vi "Main Page.vi"(8 "error in (no error)":errorcluster, 11 "Node Ptr":T1 format="%.0x") -> (0 "error out":errorcluster)   [LabVIEW 2020, in "G5 Regatron Custom Device System Explorer.lvlib"]
uses:
  G5 Regatron Custom Device System Explorer.lvlib
  <vilib>/NI VeriStand/Custom Device API/Custom Device Item Ref.ctl
  Shared/Constants.vi
  <vilib>/NI VeriStand/Custom Device API/Set Item Property (String).vi
  <vilib>/NI VeriStand/Custom Device API/Get Item Property (String).vi
  <vilib>/NI VeriStand/Custom Device API/Custom Device API.lvlib
  Shared/G5 Regatron Custom Device Shared.lvlib
panel:
  in  "Regatron IP Address":string="000.000.000.000"
  out "Version":string
  in  "SHDocVw.IWebBrowser":refnum<k7>(container)
  in  "Specific Header":cluster{"Section Name":string}={"Section Name"="Custom Device Item Settings"}
  in  "General Header":cluster{"Section Name":string}={"Section Name"="General Custom Device Settings"}
  in  "Description":string
  in  "Name":string
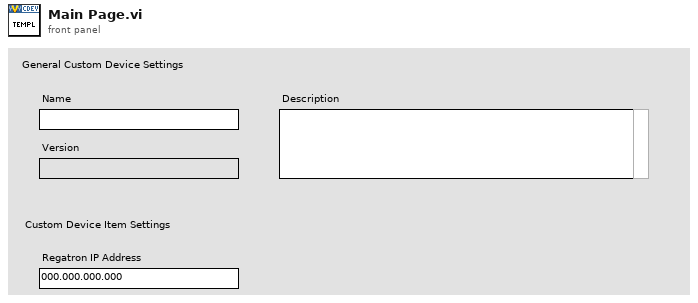
[diagram p1: front panel]
types:
  T1 = typedef "Custom Device API.lvlib/Custom Device Item Ref.ctl" = u64
  T2 = typedef "Custom Device API.lvlib/Custom Device Item Info.ctl" = cluster{"Name":string, "Is Channel":bool, "GUID":string, "Is Waveform":bool}
  T3 = typedef "Custom Device API.lvlib/Custom Device Commands.ctl" = enum16{"Default", "Item renamed", "Shutdown", "Dynamic button pressed"}
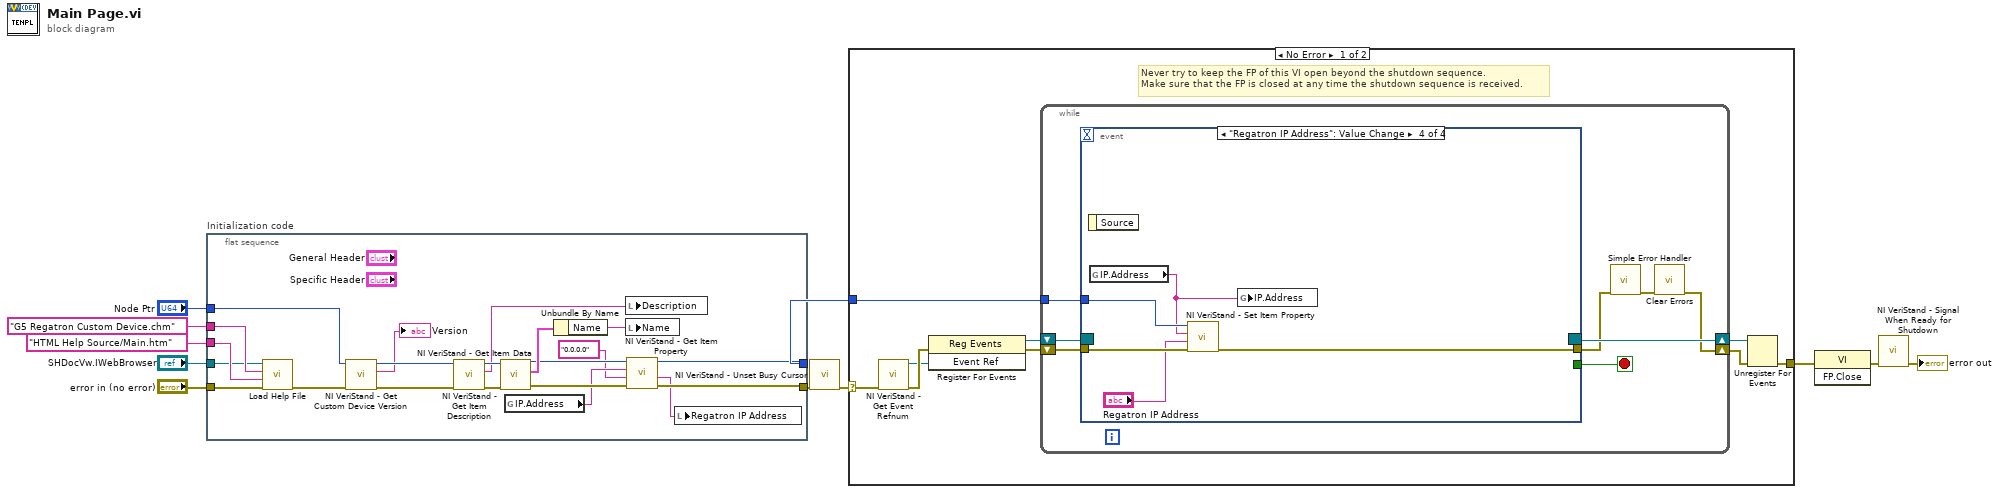
[diagram p0: block diagram]
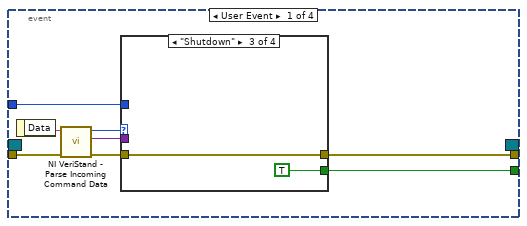
[diagram p2: hidden frame]
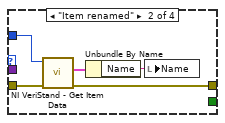
[diagram p4: hidden frame]
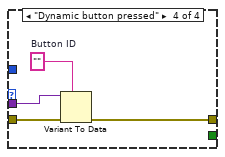
[diagram p5: hidden frame]
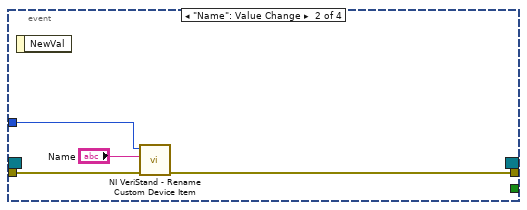
[diagram p6: hidden frame]
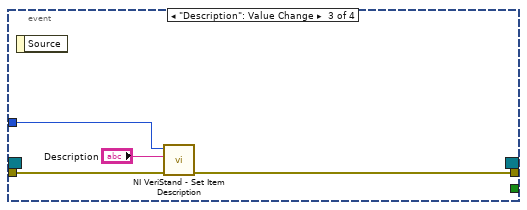
[diagram p7: hidden frame]
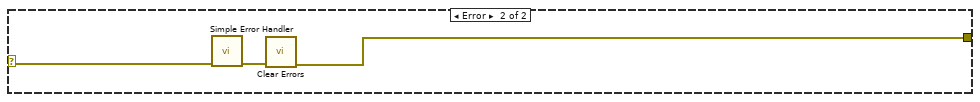
[diagram p8: hidden frame]
diagram:
  n1 = flat-sequence "Initialization code" {
    tunnel: "error in (no error)" -> [w23]
    tunnel: "Node Ptr" -> [w29]
    tunnel: [w16] -> w7
    tunnel: [w17] -> w4
    tunnel: "SHDocVw.IWebBrowser" -> [w19]
    tunnel: "HTML Help Source/Main.htm" ("HTML File") -> [w20]
    tunnel: "G5 Regatron Custom Device.chm" ("CD_CHM_FileName") -> [w21]
    frame #0 {
      n2 = call "Load Help File.vi"("error in (no error)"=w23, "HTML File to Load"=w20, "Main CHM File"=w21, "Browser"=w19) -> ("error out"=w22:errorcluster)  [unwired: 7 in]
      n3 = call <vilib>:"NI VeriStand - Get Custom Device Version.vi"("error in (no error)"=w22, "Device Ref in"=w29) -> ("error out"=w28:errorcluster, "Value"=→"Version":string, "Device Ref out"=w27:T1)  [unwired: 7 in]
      n4 = call <vilib>:"NI VeriStand - Get Item Description.vi"("error in (no error)"=w28, "Item Ref in"=w27) -> ("error out"=w31:errorcluster, "Description"=w24:string, "Item Ref out"=w32:T1)  [unwired: 7 out]
      n5 = call <vilib>:"NI VeriStand - Get Item Data.vi"("error in (no error)"=w31, "Item Ref in"=w32) -> ("error out"=w15:errorcluster, "Item Info"=w30:T2, "Item Ref out"=w18:T1)  [unwired: 7 out]
      n6 = global read "Constants.vi" "IP.Address"() -> (w14:string)
      n7 = Unbundle By Name(w30) -> ("Name"=w25:string)
      n8 = local write "Description"(w24) -> ()
      n9 = local write "Name"(w25) -> ()
      n10 = call-poly <vilib>:"NI VeriStand - Get Item Property.vi"("error in (no error)"=w15, "Default Value"="0.0.0.0", "Property Name"=w14, "Item Ref in"=w18) -> ("error out"=w16:errorcluster, "Value"=w12:string, "Item Ref out"=w17:T1)  [unwired: 4 in, 1 out]
      n11 = local write "Regatron IP Address"(w12) -> ()
    }
  }
  n12 = call <vilib>:"NI VeriStand - Unset Busy Cursor.vi"("error in (no error)"=w7) -> ("error out"=w6:errorcluster)  [unwired: 10 out]
  n13 = case shown="No Error" w6 {
    selector: w6 -> [w33 w85]
    tunnel: [w38 w83] -> w11
    tunnel: w4 -> [w34 _]
    frame No Error {
      # "Never try to keep the FP of this VI open beyond the shutdown sequence.\nMake sure that the FP is closed at any time the shutdown sequence is received."
      n14 = call <vilib>:"NI VeriStand - Get Event Refnum.vi"("error in (no error)"=w33) -> ("error out"=w41:errorcluster, "Event Ref"=w37:refnum<user-event>)  [unwired: 9 out]
      n15 = register-events(error in=w41, w37) -> (reference out=w35:refnum<event-registration>, error out=w36:errorcluster)  [unwired: 1 in]
      n16 = while {
        tunnel: w34 -> [w45]
        shift-right: [w42] -> w39
        shift-left: w36 -> [w48]
        shift-right: [w49] -> w40
        shift-left: w35 -> [w47]
        stop <- w46 stop-if-true
        n17 = event shown="[3] \"Regatron IP Address\": Value Change" {
          selector: w47 -> [_ _ _ _]
          dyn-events: [_ _ _ _] -> w49
          timeout: _ -> [_ _ _ _]
          tunnel: w48 -> [w57 w73 w76 w81]
          tunnel: [w53 _ _ _] -> w46
          tunnel: [w52 w72 w75 w79] -> w44
          tunnel: w45 -> [w51 w71 w77 w82]
          event User Event {
            n18 = event-data() -> ("Data"=w56:string)  [unwired: 1 out]
            n19 = call <vilib>:"NI VeriStand - Parse Incoming Command Data.vi"("error in (no error)"=w57, "Incoming data"=w56) -> ("error out"=w55:errorcluster, "Outgoing data"=w50:variant, "Action"=w54:T3)  [unwired: 7 out]
            n20 = case shown="\"Shutdown\"" w54 {
              tunnel: w55 -> [w58 w63 w64 w69]
              tunnel: [_ _ TRUE _] -> w53
              tunnel: [w58 w60 w64 w66] -> w52
              tunnel: w51 -> [_ w62 _ _]
              tunnel: w50 -> [_ _ _ w68]
              frame "Default", Default {
              }
              frame "Item renamed" {
                n21 = call <vilib>:"NI VeriStand - Get Item Data.vi"("error in (no error)"=w63, "Item Ref in"=w62) -> ("error out"=w60:errorcluster, "Item Info"=w61:T2)  [unwired: 8 out]
                n22 = Unbundle By Name(w61) -> ("Name"=w59:string)
                n23 = local write "Name"(w59) -> ()
              }
              frame "Shutdown" {
              }
              frame "Dynamic button pressed" {
                w67 = ""  # Button ID
                n24 = Variant To Data(error in=w69, type=w67, Variant=w68) -> (error out=w66:errorcluster)  [unwired: 1 out]
              }
            }
          }
          event "Name": Value Change {
            n25 = event-data() -> ()  [unwired: 2 out]
            n26 = call <vilib>:"NI VeriStand - Rename Custom Device Item.vi"("error in (no error)"=w73, "New Name"="Name", "Item Ref in"=w71) -> ("error out"=w72:errorcluster)  [unwired: 1 in, 7 out]
          }
          event "Description": Value Change {
            n27 = event-data() -> ()  [unwired: 2 out]
            n28 = call <vilib>:"NI VeriStand - Set Item Description.vi"("error in (no error)"=w76, "Description"="Description", "Item Ref in"=w77) -> ("error out"=w75:errorcluster)  [unwired: 8 out]
          }
          event "Regatron IP Address": Value Change {
            n29 = event-data() -> ()  [unwired: 2 out]
            n30 = global read "Constants.vi" "IP.Address"() -> (w78:string)
            n31 = call-poly <vilib>:"NI VeriStand - Set Item Property.vi"("error in (no error)"=w81, "Value"="Regatron IP Address", "Property Name"=w78, "Item Ref in"=w82) -> ("error out"=w79:errorcluster)  [unwired: 5 in, 2 out]
            n32 = global write "Constants.vi" "IP.Address"(w78) -> ()
          }
        }
        n33 = call <vilib>:"Simple Error Handler.vi"("error in (no error)"=w44) -> ("error out"=w43:errorcluster)  [unwired: 1 in, 7 out]
        n34 = call <vilib>:"Clear Errors.vi"("error in (no error)"=w43) -> ("error out"=w42:errorcluster)  [unwired: 1 in, 5 out]
      }
      n35 = Unregister For Events(event registration refnum=w40, error in=w39) -> (error out=w38:errorcluster)
    }
    frame Error {
      n36 = call <vilib>:"Simple Error Handler.vi"("error in (no error)"=w85) -> ("error out"=w84:errorcluster)  [unwired: 1 in, 7 out]
      n37 = call <vilib>:"Clear Errors.vi"("error in (no error)"=w84) -> ("error out"=w83:errorcluster)  [unwired: 1 in, 5 out]
    }
  }
  n38 = invoke class="VI" method="FP.Close"(error in=w11) -> (error out=w10:errorcluster)  [unwired: 2 in, 2 out]
  n39 = call <vilib>:"NI VeriStand - Signal When Ready for Shutdown.vi"("error in (no error)"=w10) -> ("error out"=→"error out":errorcluster)  [unwired: 10 out]
